vi "CRYAPI WSYSTEM LIB HIGHT.vi"(8 "sOption":string, 9 "sData":string, 10 "nData":i32, 11 "sAction":string) -> (0 "nData_Out":i32, 3 "tFrame_Out":T2)   [LabVIEW 2013]
uses:
  <vilib>/Utility/miscctls.llb/LVRectTypeDef.ctl
  DataView/VIEW/CRYView Global.vi
  CRYMain Sub Window Global.vi
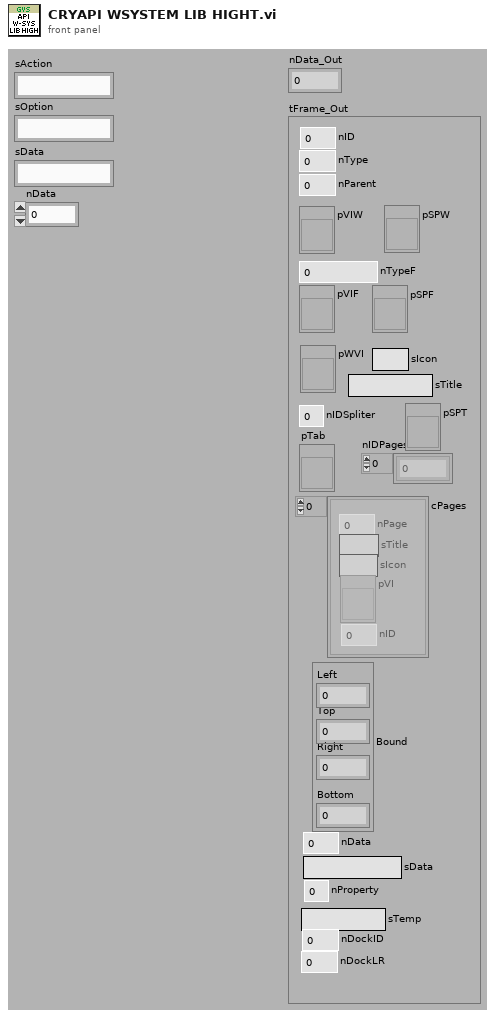
[diagram p1: front panel]
types:
  T1 = typedef "LVRectTypeDef.ctl" = cluster{"Left":i16, "Top":i16, "Right":i16, "Bottom":i16}
  T2 = cluster{"nType":i32, "nParent":i32, "pVIW":refnum<vi>, "pSPW":refnum<vi>, "nTypeF":i32, "pVIF":refnum<vi>, "pSPF":refnum<vi>, "nIDSpliter":i32, "nProperty":i32, "Bound":T1, "nID":i32, "nData":i32, "sData":string, "pWVI":refnum<vi>, "sTitle":string, "cPages":cluster{"nPage":i32, "sTitle":string, "sIcon":string, "pVI":refnum<vi>, "nID":i32}[], "pTab":refnum<vi>, "nIDPages":i32[], "pSPT":refnum<vi>, "sTemp":string, "nDockID":i32, "nDockLR":i32, "sIcon":string}
  T3 = cluster{"sAction":string, "sType":string, "sQueueName":string, "sGraphName":string, "sData":string, "nData":i32, "pVIRef":refnum<vi>, "pSPRef":refnum<vi>}
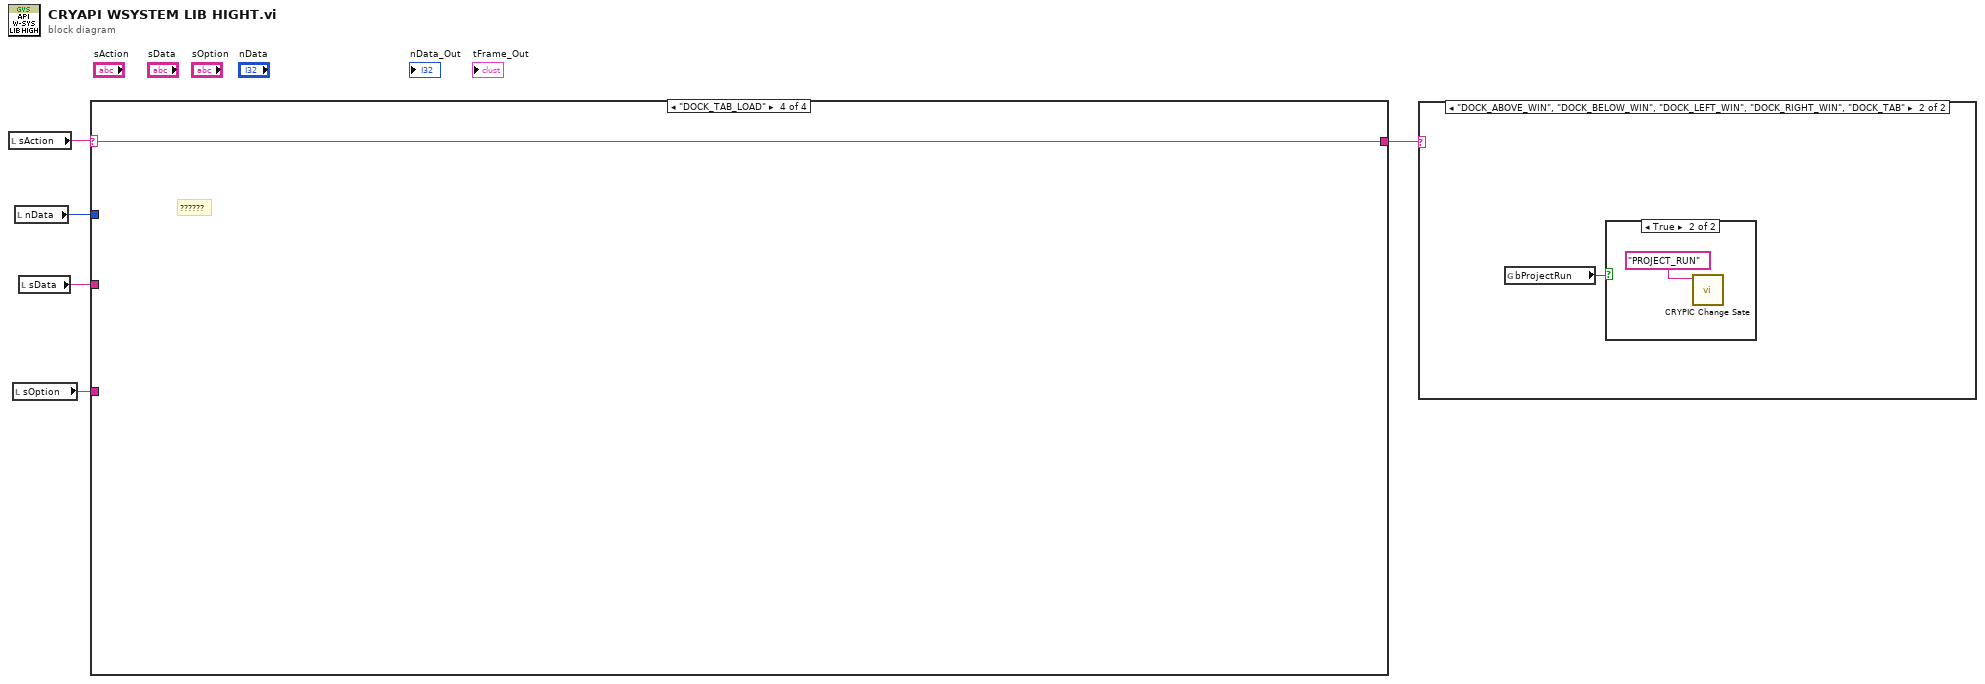
[diagram p0: block diagram]
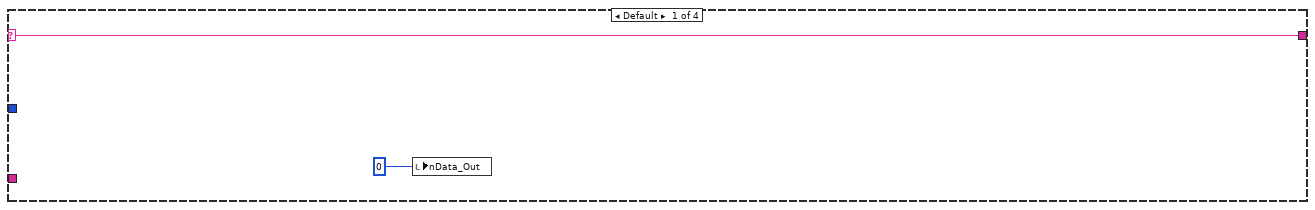
[diagram p4: hidden frame]
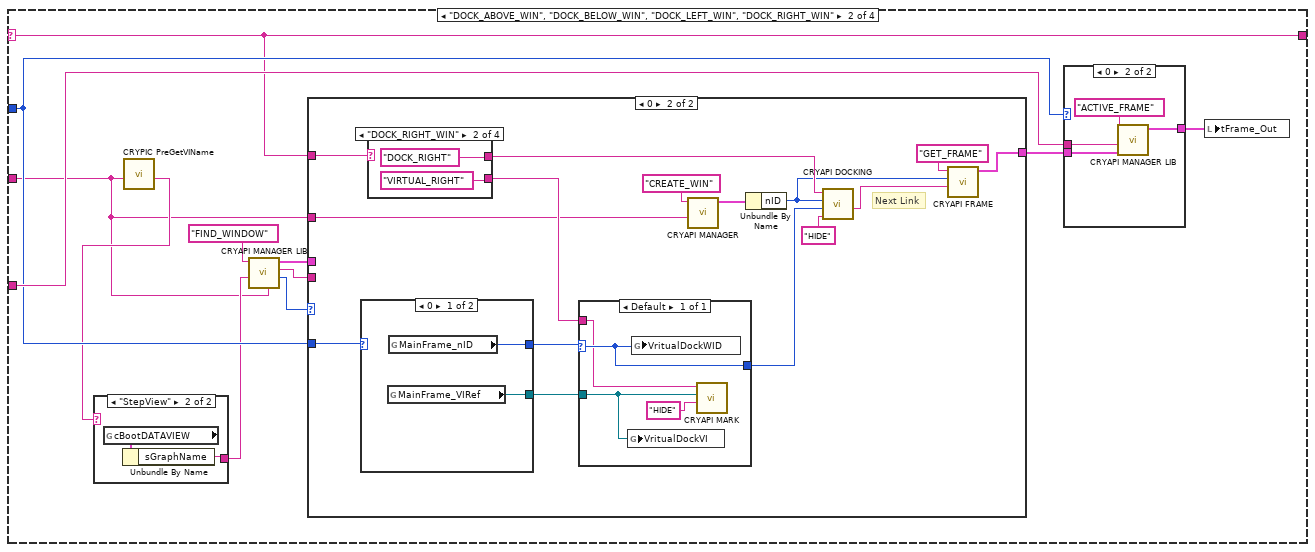
[diagram p5: hidden frame]
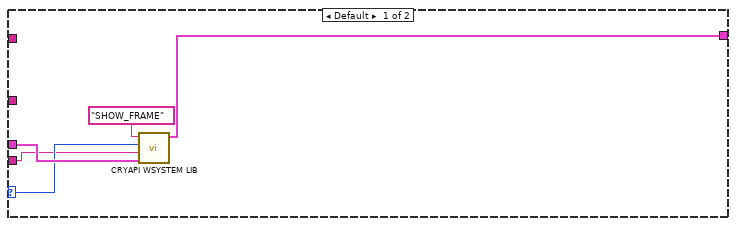
[diagram p8: hidden frame]
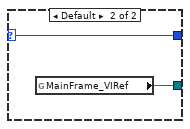
[diagram p9: hidden frame]
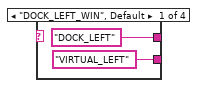
[diagram p10: hidden frame]
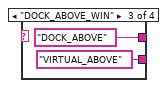
[diagram p11: hidden frame]
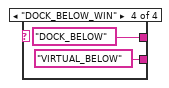
[diagram p12: hidden frame]
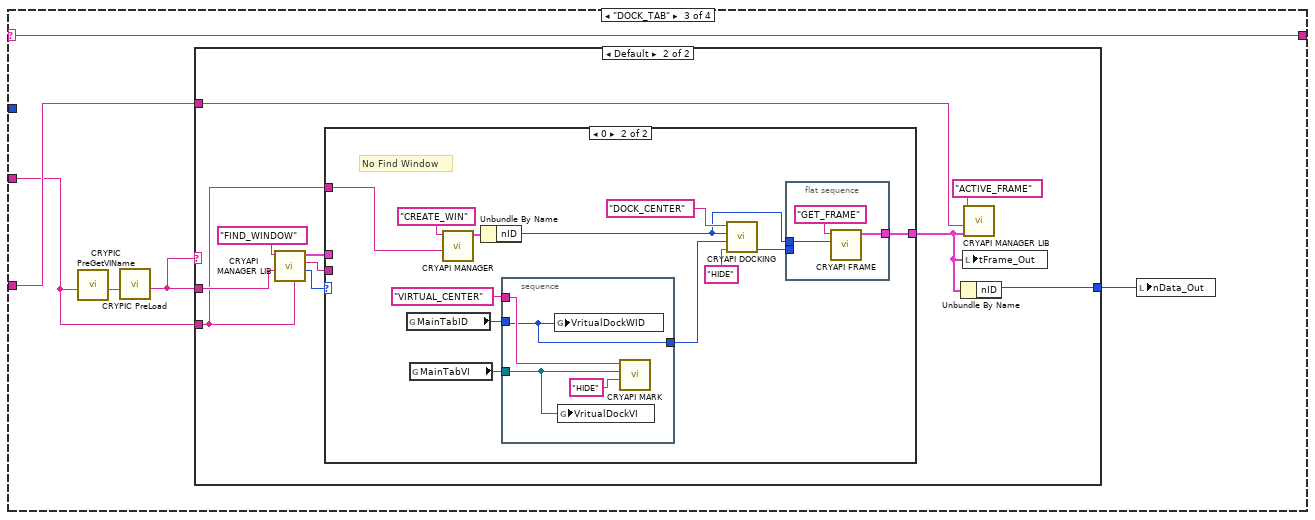
[diagram p13: hidden frame]
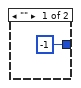
[diagram p14: hidden frame]
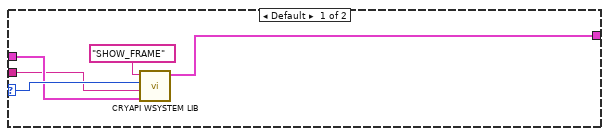
[diagram p15: hidden frame]
diagram:
  n1 = local read "sAction"() -> (w5:string)
  n2 = local read "sOption"() -> (w2:string)
  n3 = local read "nData"() -> (w3:i32)
  n4 = local read "sData"() -> (w4:string)
  n5 = case shown="\"DOCK_TAB_LOAD\"" w5 {
    selector: w5 -> [w6 w8 w64 w105]
    tunnel: w4 -> [_ w9 w68 _]
    tunnel: w3 -> [_ w12 _ _]
    tunnel: w2 -> [_ w14 w69 _]
    tunnel: [w6 w8 w64 w105] -> w1
    frame Default {
      n6 = local write "nData_Out"(0 ("nData_Out")) -> ()
    }
    frame "DOCK_ABOVE_WIN", "DOCK_BELOW_WIN", "DOCK_LEFT_WIN", "DOCK_RIGHT_WIN" {
      n7 = call "CRYPIC PreGetVIName.vi"("sVIName"=w9) -> ("sVIName_Out"=w10:string)  [unwired: 9 in, 1 out]
      n8 = case shown="\"StepView\"" w10 {
        selector: w10 -> [w20 _]
        tunnel: [w20 w21] -> w11
        frame Default {
        }
        frame "StepView" {
          n9 = global read "CRYView Global.vi" "cBootDATAVIEW"() -> (w22:T3)
          n10 = Unbundle By Name(w22) -> ("sGraphName"=w21:string)
        }
      }
      n11 = call "CRYAPI MANAGER LIB.vi"("sOption"=w9, "sData"=w11, "sAction"="FIND_WINDOW") -> ("nData_Out"=w16:i32, "sData_Out"=w19:string, "tFrame_Out"=w18:T2)  [unwired: 6 in]
      n12 = case shown="0" w16 {
        selector: w16 -> [w30 _]
        tunnel: w8 -> [_ w46]
        tunnel: w9 -> [_ w39]
        tunnel: [w29 w36] -> w17
        tunnel: w18 -> [w31 _]
        tunnel: w19 -> [w28 _]
        tunnel: w12 -> [_ w35]
        frame Default {
          n13 = call "CRYAPI WSYSTEM LIB.vi"("tFrame"=w31, "sData"=w28, "nData"=w30, "sAction"="SHOW_FRAME") -> ("tFrame_Out"=w29:T2)  [unwired: 7 out]
        }
        frame 0 {
          # "Next Link"
          n14 = case shown="0" w35 {
            selector: w35 -> [_ w50]
            tunnel: [w49 w50] -> w44
            tunnel: [w48 w51] -> w42
            frame 0 {
              n15 = global read "CRYMain Sub Window Global.vi" "MainFrame_VIRef"() -> (w48:refnum<vi>)
              n16 = global read "CRYMain Sub Window Global.vi" "MainFrame_nID"() -> (w49:i32)
            }
            frame Default {
              n17 = global read "CRYMain Sub Window Global.vi" "MainFrame_VIRef"() -> (w51:refnum<vi>)
            }
          }
          n18 = case shown="\"DOCK_RIGHT_WIN\"" w46 {
            tunnel: ["DOCK_LEFT" "DOCK_RIGHT" "DOCK_ABOVE" "DOCK_BELOW"] -> w45
            tunnel: ["VIRTUAL_LEFT" "VIRTUAL_RIGHT" "VIRTUAL_ABOVE" "VIRTUAL_BELOW"] -> w41
            frame "DOCK_LEFT_WIN", Default {
            }
            frame "DOCK_RIGHT_WIN" {
            }
            frame "DOCK_ABOVE_WIN" {
            }
            frame "DOCK_BELOW_WIN" {
            }
          }
          n19 = case shown="Default" w44 {
            selector: w44 -> [w55]
            tunnel: [w55] -> w43
            tunnel: w42 -> [w53]
            tunnel: w41 -> [w52]
            frame Default {
              n20 = global write "CRYMain Sub Window Global.vi" "VritualDockVI"(w53) -> ()
              n21 = global write "CRYMain Sub Window Global.vi" "VritualDockWID"(w55) -> ()
              n22 = call "CRYAPI MARK.vi"("sAction"=w52, "mVritual_VIRef"=w53, "sData"="HIDE") -> ()  [unwired: 1 in, 7 out]
            }
          }
          n23 = call "CRYAPI MANAGER.vi"("sData"=w39, "sAction"="CREATE_WIN") -> ("tFrame_Out"=w38:T2)  [unwired: 3 in, 6 out]
          n24 = Unbundle By Name(w38) -> ("nID"=w37:i32)
          n25 = call "CRYAPI DOCKING.vi"("sData"="HIDE", "nDWinID"=w43, "nSWinID"=w37, "sAction"=w45) -> ("sData_Out"=w33:string)  [unwired: 7 out]
          n26 = call "CRYAPI FRAME.vi"("sData"=w33, "nData"=w37, "sAction"="GET_FRAME") -> ("tFrame_Out"=w36:T2)  [unwired: 3 in, 5 out]
        }
      }
      n27 = case shown="0" w12 {
        tunnel: w17 -> [w23 w27]
        tunnel: w14 -> [_ w25]
        tunnel: [w23 w24] -> w13
        frame Default {
        }
        frame 0 {
          n28 = call "CRYAPI MANAGER LIB.vi"("tFrame"=w27, "sData"=w25, "sAction"="ACTIVE_FRAME") -> ("tFrame_Out"=w24:T2)  [unwired: 6 in, 2 out]
        }
      }
      n29 = local write "tFrame_Out"(w13) -> ()
    }
    frame "DOCK_TAB" {
      n30 = call "CRYPIC PreGetVIName.vi"("sVIName"=w68) -> ("sVIName_Out"=w67:string)  [unwired: 9 in, 1 out]
      n31 = call "CRYPIC PreLoad.vi"("sVIName"=w67) -> ("sVITitle_Out"=w66:string)  [unwired: 10 in]
      n32 = case shown="Default" w66 {
        tunnel: w69 -> [_ w76]
        tunnel: w66 -> [_ w73]
        tunnel: w68 -> [_ w72]
        tunnel: [-1 ("nID") w71] -> w65
        frame "" {
        }
        frame Default {
          n33 = call "CRYAPI MANAGER LIB.vi"("sOption"=w72, "sData"=w73, "sAction"="FIND_WINDOW") -> ("nData_Out"=w77:i32, "sData_Out"=w80:string, "tFrame_Out"=w78:T2)  [unwired: 6 in]
          n34 = case shown="0" w77 {
            selector: w77 -> [w84 _]
            tunnel: w72 -> [_ w90]
            tunnel: w78 -> [w83 _]
            tunnel: [w82 w88] -> w75
            tunnel: w80 -> [w81 _]
            frame Default {
              n35 = call "CRYAPI WSYSTEM LIB.vi"("tFrame"=w83, "sData"=w81, "nData"=w84, "sAction"="SHOW_FRAME") -> ("tFrame_Out"=w82:T2)  [unwired: 7 out]
            }
            frame 0 {
              # "No Find Window"
              n36 = global read "CRYMain Sub Window Global.vi" "MainTabID"() -> (w87:i32)
              n37 = global read "CRYMain Sub Window Global.vi" "MainTabVI"() -> (w93:refnum<vi>)
              n38 = call "CRYAPI MANAGER.vi"("sData"=w90, "sAction"="CREATE_WIN") -> ("tFrame_Out"=w95:T2)  [unwired: 3 in, 6 out]
              n39 = Unbundle By Name(w95) -> ("nID"=w89:i32)
              n40 = stacked-sequence {
                tunnel: [w101] -> w94
                tunnel: w93 -> [w103]
                tunnel: "VIRTUAL_CENTER" -> [w102]
                tunnel: w87 -> [w101]
                frame #0 {
                  n41 = global write "CRYMain Sub Window Global.vi" "VritualDockWID"(w101) -> ()
                  n42 = global write "CRYMain Sub Window Global.vi" "VritualDockVI"(w103) -> ()
                  n43 = call "CRYAPI MARK.vi"("sAction"=w102, "mVritual_VIRef"=w103, "sData"="HIDE") -> ()  [unwired: 1 in, 7 out]
                }
              }
              n44 = call "CRYAPI DOCKING.vi"("sData"="HIDE", "nDWinID"=w94, "nSWinID"=w89, "sAction"="DOCK_CENTER") -> ("nData_Out"=w86:i32)  [unwired: 7 out]
              n45 = flat-sequence {
                tunnel: w89 -> [w100]
                tunnel: [w99] -> w88
                tunnel: w86 -> [_]
                frame #0 {
                  n46 = call "CRYAPI FRAME.vi"("nData"=w100, "sAction"="GET_FRAME") -> ("tFrame_Out"=w99:T2)  [unwired: 4 in, 5 out]
                }
              }
            }
          }
          n47 = Unbundle By Name(w75) -> ("nID"=w71:i32)
          n48 = local write "tFrame_Out"(w75) -> ()
          n49 = call "CRYAPI MANAGER LIB.vi"("tFrame"=w75, "sData"=w76, "sAction"="ACTIVE_FRAME") -> ()  [unwired: 6 in, 3 out]
        }
      }
      n50 = local write "nData_Out"(w65) -> ()
    }
    frame "DOCK_TAB_LOAD" {
      # "??????"
    }
  }
  n51 = case shown="\"DOCK_ABOVE_WIN\", \"DOCK_BELOW_WIN\", \"DOCK_LEFT_WIN\", \"DOCK_RIGHT_WIN\", \"DOCK_TAB\"" w1 {
    frame "False", Default {
    }
    frame "DOCK_ABOVE_WIN", "DOCK_BELOW_WIN", "DOCK_LEFT_WIN", "DOCK_RIGHT_WIN", "DOCK_TAB" {
      n52 = global read "CRYMain Sub Window Global.vi" "bProjectRun"() -> (w106:bool)
      n53 = case shown="True" w106 {
        frame False {
        }
        frame True {
          n54 = call "CRYPIC Change Sate.vi"("sAction"="PROJECT_RUN") -> ()  [unwired: 10 in, 1 out]
        }
      }
    }
  }
